vi "novoGoleiroPosicionarseAtrasBola.vi"(8 "Goleiro.X_padrao":dbl, 9 "balls":T1[](array[typedef]), 10 "Robot in":T2, 11 "IA State":T7={"our_robots"=[], "enemy_robots"=[], "balls"=[], "geometry"={"field_length"=0, "field_width"=0, "goal_width"=0, "goal_depth"=0, "center_circle_radius"=0, "defense_width"=0, "defense_depth"=0, "free_kick_from_defense_dist"=0, "penalty_spot_from_field_line_dist"=0, "penalty_line_from_spot_dist"=0, "half_moon_depth"=0, "half_moon_width"=0}, "IA Judge"={"stage"="", "command"="", "our_goalie_id"=0.0, "enemy_goalie_id"=0.0, "command enum"=enum."Halt", "Time"=enum."Azul"}, "Received Timestamp"=timestamp(0 s since 1904-01-01), "Events"={"Touch"=FALSE, "id touch"=0.0, "Ball out of \nVision"=FALSE, "Ball inside \nGoalie area"=FALSE, "Robot not responding"=FALSE, "Robots responding status"=[1.0, 1.0, 1.0, 1.0, 1.0, 1.0], "Enemy Ball \nPossession"=FALSE, "Id ini Possession"=0.0, "Ball Possesion"=FALSE, "Id Possesion"=0.0, "Ball at\nour goal side"=FALSE, "Ball at\ntouchline"=FALSE, "Ball at\nenemy goal side"=FALSE}}) -> (3 "Cluster de saída":T2)   [LabVIEW 2018]
uses:
  Core/AI Input.ctl
  Desktop/VSS pra teste willrich/VSS/Core/AI Robot.ctl
  Desktop/VSS pra teste willrich/VSS/Intel/Functions Enum.ctl
  Desktop/VSS pra teste willrich/VSS/Intel/AttackerStates.ctl
  Desktop/VSS pra teste willrich/VSS/Path Planning/RRT/PathDests.ctl
  Desktop/VSS pra teste willrich/VSS/Path Planning/RRT/PathDest.ctl
  Core/AI Ball.ctl
  Core/Field Size.ctl
  Core/AI Judge.ctl
  Intel/Command Enum.ctl
  Util/Events/Events.ctl
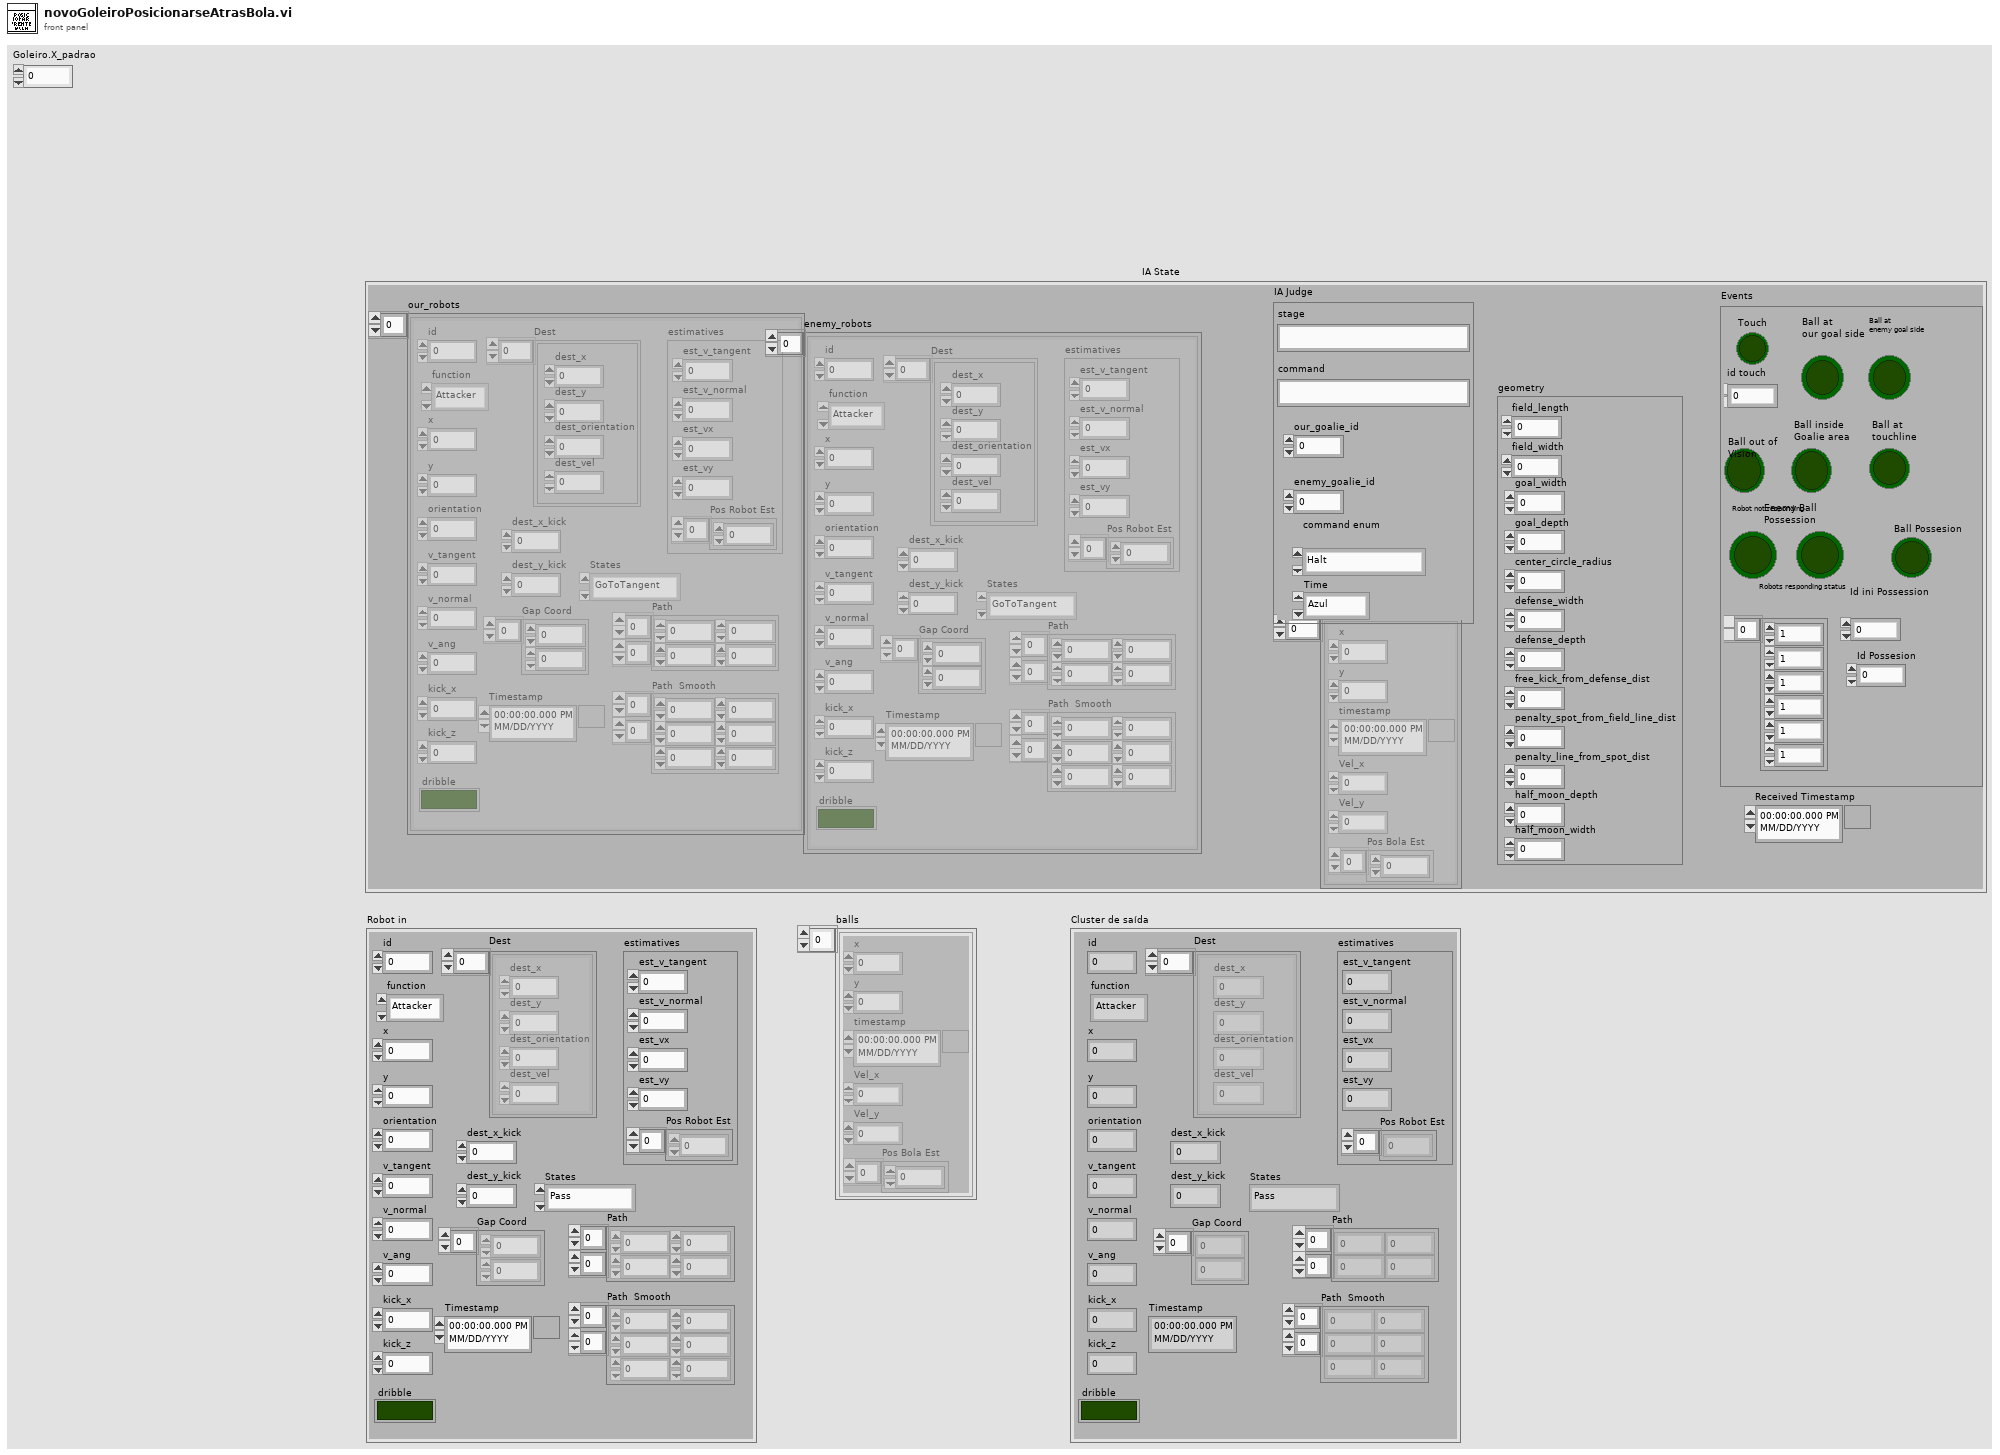
[diagram p1: front panel]
types:
  T1 = typedef "AI Ball.ctl" = cluster{"x":dbl, "y":dbl, "timestamp":timestamp, "Vel_x":dbl, "Vel_y":dbl, "Pos Bola Est":dbl[]}
  T2 = typedef "AI Robot.ctl" = cluster{"id":u32, "function":T3, "x":dbl, "y":dbl, "orientation":dbl, "v_tangent":dbl, "v_normal":dbl, "v_ang":dbl, "kick_x":dbl, "kick_z":dbl, "dribble":bool, "Timestamp":timestamp, "estimatives":cluster{"est_v_tangent":dbl, "est_v_normal":dbl, "est_vx":dbl, "est_vy":dbl, "Pos Robot Est":dbl[]}, "dest_x_kick":dbl, "dest_y_kick":dbl, "Gap Coord":dbl[], "States":T4, "Path ":dbl[][], "Path  Smooth":dbl[][], "Dest":T5}
  T3 = typedef "Functions Enum.ctl" = enum16{"Attacker", "Goalie", "Defender", "Striker", "Goto 0", "Dummy", "Kicker", "ZigZag"}
  T4 = typedef "AttackerStates.ctl" = enum16{"Pass", "GoToTangent", "BallGetting", "GoToKick", "Rotate anti-clockwise", "Rotate Clockwise", ""}
  T5 = typedef "PathDests.ctl" = T6[]
  T6 = typedef "PathDest.ctl" = cluster{"dest_x":dbl, "dest_y":dbl, "dest_orientation":dbl, "dest_vel":dbl}
  T7 = typedef "AI Input.ctl" = cluster{"our_robots":T2[], "enemy_robots":T2[], "balls":T1[], "geometry":T8, "IA Judge":T9, "Received Timestamp":timestamp, "Events":T11}
  T8 = typedef "Field Size.ctl" = cluster{"field_length":u32, "field_width":u32, "goal_width":u32, "goal_depth":u32, "center_circle_radius":u32, "defense_width":u32, "defense_depth":u32, "free_kick_from_defense_dist":u32, "penalty_spot_from_field_line_dist":u32, "penalty_line_from_spot_dist":u32, "half_moon_depth":u32, "half_moon_width":u32}
  T9 = typedef "AI Judge.ctl" = cluster{"stage":string, "command":string, "our_goalie_id":dbl, "enemy_goalie_id":dbl, "command enum":T10, "Time":enum16{"Azul", "Amarelo"}}
  T10 = typedef "Command Enum.ctl" = enum16{"Halt", "Stop", "Force Start", "PKA Normal Start", "Prepare Kickoff Ally", "PKE Normal Start", "Prepare Kickoff Enemy", "Prepare Penalty Ally", "PPA Normal Start", "Prepare Penalty Enemy", "PPE Normal Start", "Ball Placement Enemy Up", "Ball Placement Enemy Down", "Ball Placement Ally Up", "Ball Placement Ally Mid", "Ball Placement Ally Down", "Indirect Free Enemy", "Indirect Free Ally", "Timeout Enemy", "Timeout Ally", "Goal Enemy", "Goal Ally", "Normal Half Time", "Extra Time Break", "Extra Half Time", "None", "Post Game"}
  T11 = typedef "Events.ctl" = cluster{"Touch":bool, "id touch":dbl, "Ball out of \nVision":bool, "Ball inside \nGoalie area":bool, "Robot not responding":bool, "Robots responding status":dbl[], "Enemy Ball \nPossession":bool, "Id ini Possession":dbl, "Ball Possesion":bool, "Id Possesion":dbl, "Ball at\nour goal side":bool, "Ball at\ntouchline":bool, "Ball at\nenemy goal side":bool}
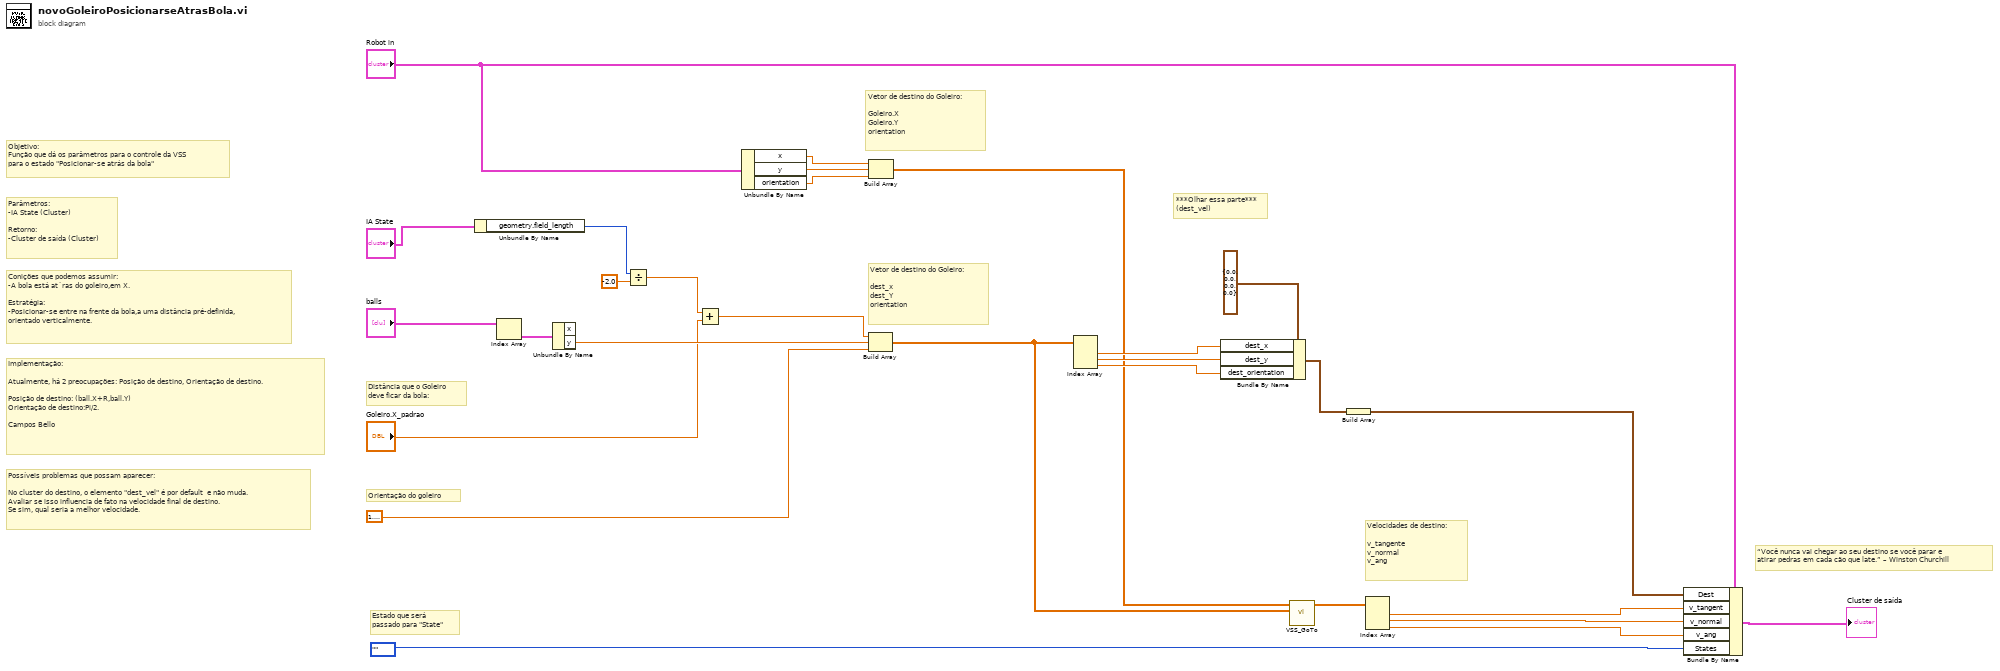
[diagram p0: block diagram]
diagram:
  # "Vetor de destino do Goleiro:\n\nGoleiro.X\nGoleiro.Y\norientation"
  # "Vetor de destino do Goleiro:\n\ndest_x\ndest_Y\norientation"
  # "Orientação do goleiro"
  # "“Você nunca vai chegar ao seu destino se você parar e\natirar pedras em cada cão que late.” – Winston Churchill"
  # "Conições que podemos assumir:\n-A bola está at´ras do goleiro,em X.\n\nEstratégia:\n-Posicionar-se entre na frente da bola,a uma distância pré-definida,\norientado verticalmente."
  # "Possíveis problemas que possam aparecer:\n\nNo cluster do destino, o elemento \"dest_vel\" é por default  e não muda. \nAvaliar se isso influencia de fato na velocidade final de destino.\nSe sim, qual seria a melhor velocidade."
  # "Implementação:\n\nAtualmente, há 2 preocupações: Posição de destino, Orientação de destino.\n\nPosição de destino: (ball.X+R,ball.Y)\nOrientação de destino:Pi/2.\n\nCampos Bello"
  # "Parâmetros:\n-IA State (Cluster)\n\nRetorno:\n-Cluster de saída (Cluster)"
  # "Objetivo:\nFunção que dá os parâmetros para o controle da VSS\npara o estado \"Posicionar-se atrás da bola\""
  # "Estado que será\npassado para \"State\""
  # "Velocidades de destino:\n\nv_tangente\nv_normal\nv_ang"
  # "***Olhar essa parte***\n(dest_vel)"
  # "Distância que o Goleiro\ndeve ficar da bola:"
  n1 = Unbundle By Name("IA State") -> ("geometry.field_length"=w4:u32)
  n2 = Index Array(array="balls") -> (element=w28:T1)  [unwired: 1 in]
  n3 = Unbundle By Name(w28) -> ("y"=w17:dbl)  [unwired: 1 out]
  n4 = Divide(x=w4, y=-2.0) -> (x/y=w3:dbl)
  n5 = Add(x=w3, y="Goleiro.X_padrao") -> (x+y=w1:dbl)
  n6 = Unbundle By Name("Robot in") -> ("x"=w9:dbl, "y"=w10:dbl, "orientation"=w8:dbl)
  n7 = Build Array(w1, w17, 1.5707963267948966) -> (w12:dbl[])
  n8 = Build Array(w9, w10, w8) -> (w7:dbl[])
  n9 = Index Array(array=w12) -> (element #1=w15:dbl, element #2=w14:dbl, element #3=w13:dbl)  [unwired: 3 in]
  n10 = Bundle By Name(cluster=T6 {"dest_x"=0.0, "dest_y"=0.0, "dest_orientation"=0.0, "dest_vel"=0.0} ("element"), "dest_x"=w15, "dest_y"=w14, "dest_orientation"=w13) -> (w23:T6)
  n11 = call "VSS_GoTo.vi"("SetPoint"=w12, "Position"=w7) -> ("Output Vel"=w21:dbl[])  [unwired: 9 in]
  n12 = Build Array(w23) -> (w22:T6[])
  n13 = Index Array(array=w21) -> (element #1=w27:dbl, element #2=w26:dbl, element #3=w25:dbl)  [unwired: 3 in]
  n14 = Bundle By Name(cluster="Robot in", "Dest"=w22, "v_tangent"=w27, "v_normal"=w26, "v_ang"=w25, "States"=AttackerStates."") -> (→"Cluster de saída":T2)
